vi "LJM logger build channel setup config string.vi"(5 "delimiter (#!#)":string="#!#", 7 "Max Num Elements":i32=100, 8 "Int list":i32[](array[numeric]), 9 "Bool list":bool[](array[boolean]), 10 "String list 2":string[](array[string])=["a", "b", "c", "d", "e", "f", "g", "h", "i", "j", "k", "l", "m", "n", "o", "p", "q", "r", "s", "t", "u", "v", "w", "x", "y", "z"], 11 "String list 1":string[](array[string])=["a", "b", "c", "d", "e", "f", "g", "h", "i", "j", "k", "l", "m", "n", "o", "p", "q", "r", "s", "t", "u", "v", "w", "x", "y", "z"]) -> (0 "Int formatted":string, 1 "Bool formatted":string, 2 "String 2 formatted":string, 3 "String 1 formatted":string)   [LabVIEW 2026]
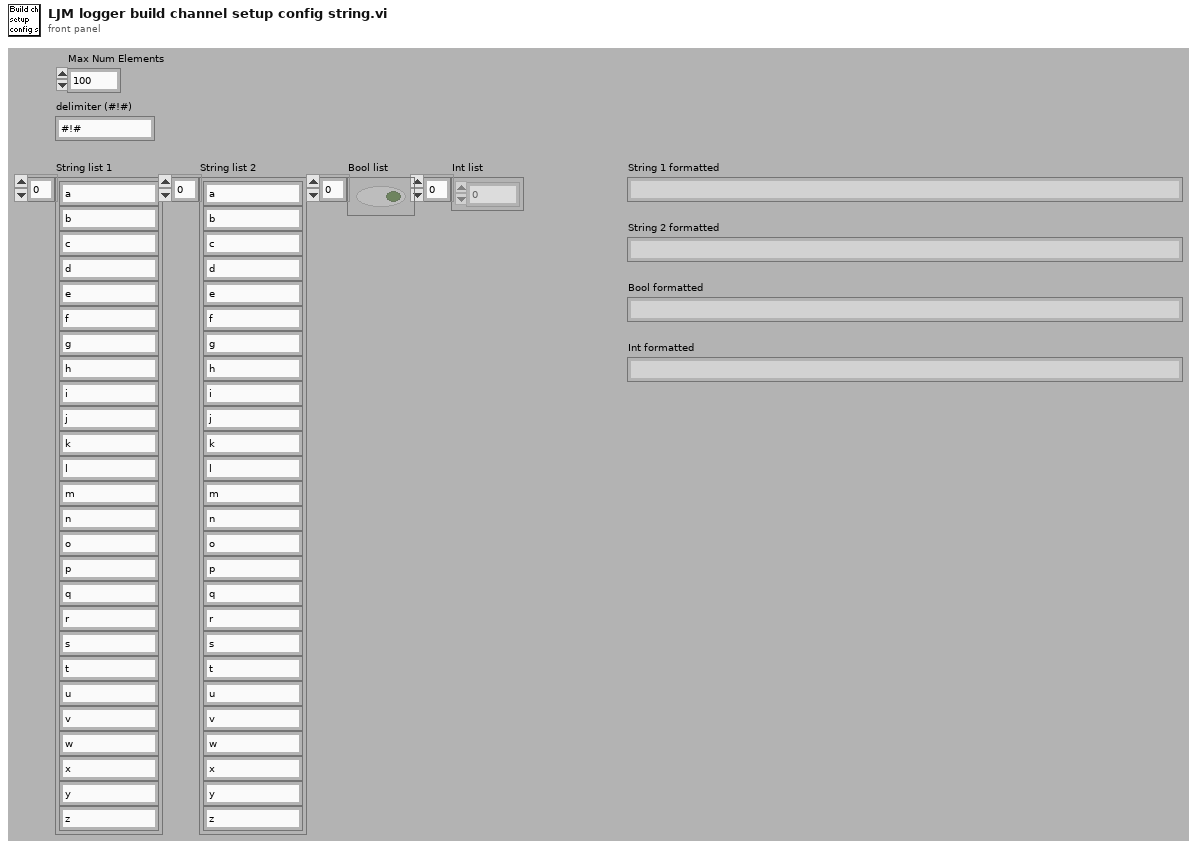
[diagram p1: front panel]
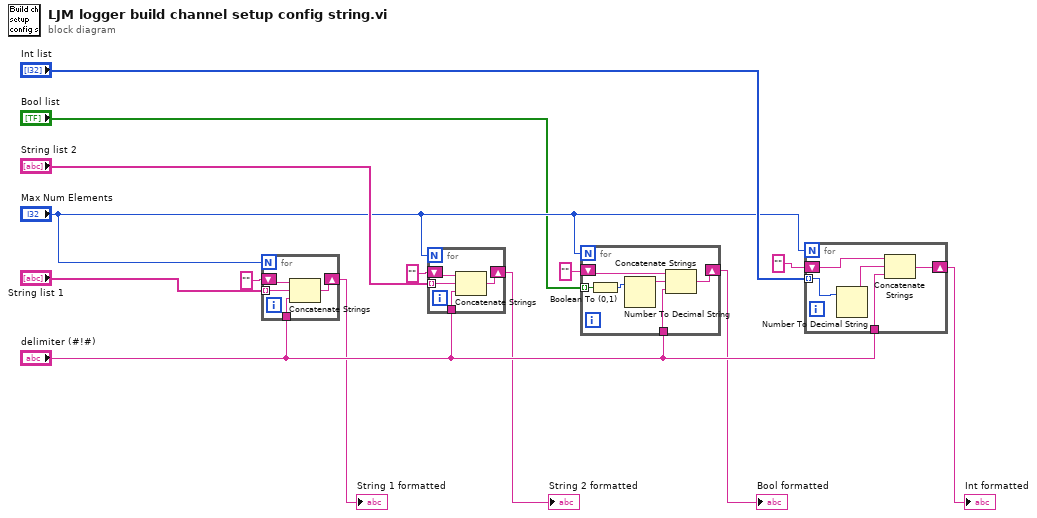
[diagram p0: block diagram]
diagram:
  n1 = for {
    N: "Max Num Elements" -> [_]
    shift-right: [w17] -> w6
    shift-left: "" -> [w18]
    tunnel: "delimiter (#!#)" -> [w16]
    tunnel: "String list 1" -> [w15] mode=indexing
    n2 = Concatenate Strings(w18, w15, w16) -> (w17:string)
  }
  "String 1 formatted" <- w6
  n3 = for {
    N: "Max Num Elements" -> [_]
    shift-right: [w21] -> w5
    shift-left: "" -> [w22]
    tunnel: "delimiter (#!#)" -> [w20]
    tunnel: "String list 2" -> [w19] mode=indexing
    n4 = Concatenate Strings(w22, w19, w20) -> (w21:string)
  }
  "String 2 formatted" <- w5
  n5 = for {
    N: "Max Num Elements" -> [_]
    shift-right: [w27] -> w4
    shift-left: "" -> [w28]
    tunnel: "delimiter (#!#)" -> [w26]
    tunnel: "Bool list" -> [w23] mode=indexing
    n6 = Boolean To (0,1)(Boolean=w23) -> (0, 1=w24:i16)
    n7 = Number To Decimal String(number=w24) -> (decimal integer string=w25:string)  [unwired: 1 in]
    n8 = Concatenate Strings(w28, w25, w26) -> (w27:string)
  }
  "Bool formatted" <- w4
  n9 = for {
    N: "Max Num Elements" -> [_]
    tunnel: "delimiter (#!#)" -> [w31]
    tunnel: "Int list" -> [w30] mode=indexing
    shift-right: [w32] -> w3
    shift-left: "" -> [w33]
    n10 = Number To Decimal String(number=w30) -> (decimal integer string=w29:string)  [unwired: 1 in]
    n11 = Concatenate Strings(w33, w29, w31) -> (w32:string)
  }
  "Int formatted" <- w3
